vi "Natural Logarithm.vi"   [LabVIEW 2024, in "NI_Matrix.lvlib"]
doc: "Computes the natural logarithm of the input matrix."
uses:
  NI_Matrix.lvlib
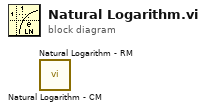
[diagram p0: block diagram]
diagram:
  n1 = call "Natural Logarithm - CM.vi"() -> ()  [unwired: 1 in, 1 out]
  n2 = call "Natural Logarithm - RM.vi"() -> ()  [unwired: 1 in, 1 out]
